vi "Arduino Analog Read Pin.vi"() -> ()   [LabVIEW 2011, in "LabVIEW Interface for Arduino.lvlib"]
doc: "An example that reads a user selectable analog input pin on the Arduino."
uses:
  <vilib>/LabVIEW Interface for Arduino/LabVIEW Interface for Arduino.lvlib
  <vilib>/LabVIEW Interface for Arduino/Type Defs/Analog Pin.ctl
panel:
  in  "Analog Pin":T1
  in  "Stop":bool
  out "Voltage":dbl(knob) scale=0.0..5.0
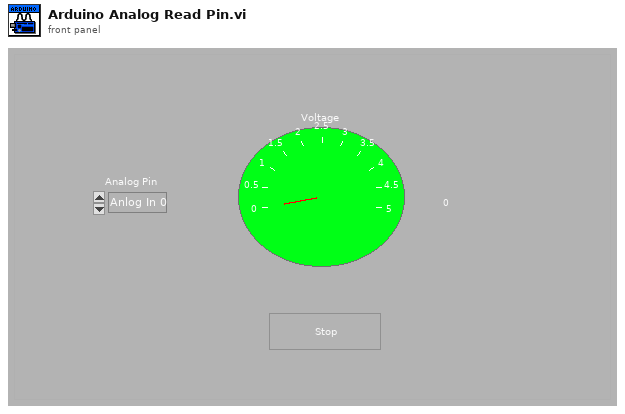
[diagram p1: front panel]
types:
  T1 = typedef "LabVIEW Interface for Arduino.lvlib/Analog Pin.ctl" = enum8{"Anlog In 0", "Anlog In 1", "Anlog In 2", "Anlog In 3", "Anlog In 4", "Anlog In 5"}
  T2 = typedef "LabVIEW Interface for Arduino.lvlib/Arduino Resource.ctl" = cluster{"VISA resource":refnum<visa-resource-name>, "Board Type":T3, "Connection Type":enum8{"USB / Serial"}, "Bytes Per Packet (15)":u8}
  T3 = typedef "LabVIEW Interface for Arduino.lvlib/Board Type.ctl" = enum16{"Uno", "Dimuelanove w/Atmega 328", "Mega 2560"}
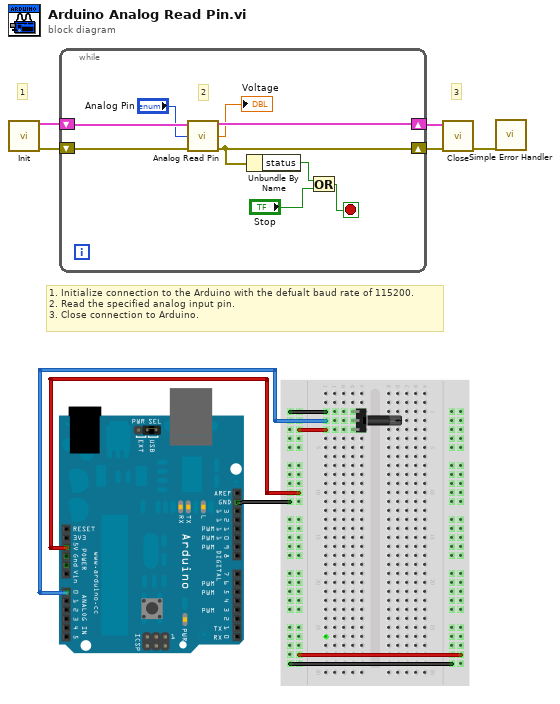
[diagram p0: block diagram]
diagram:
  # "1. Initialize connection to the Arduino with the defualt baud rate of 115200.\n2. Read the specified analog input pin.\n3. Close connection to Arduino."
  # "3"
  # "1"
  n1 = call <vilib>:"Init.vi"() -> ("Arduino Resource"=w5:T2, "error out"=w2:errorcluster)  [unwired: 18 in]
  n2 = while {
    shift-right: [w14] -> w4
    shift-left: w5 -> [w8]
    shift-right: [w12] -> w3
    shift-left: w2 -> [w7]
    stop <- w11 stop-if-true
    # "2"
    n3 = call <vilib>:"Analog Read Pin.vi"("Arduino Resource"=w8, "Analog Input Pin (0)"="Analog Pin", "error in"=w7) -> ("Arduino Resource"=w14:T2, "Voltage"=→"Voltage":dbl, "error out"=w12:errorcluster)  [unwired: 10 in]
    n4 = Unbundle By Name(w12) -> ("status"=w10:bool)
    n5 = Or(x=w10, y="Stop") -> (x .or. y?=w11:bool)
  }
  n6 = call <vilib>:"Close.vi"("Arduino Resource"=w4, "error in"=w3) -> ("error out"=w1:errorcluster)  [unwired: 13 in]
  n7 = call <vilib>:"Simple Error Handler.vi"("error in (no error)"=w1) -> ()  [unwired: 4 in, 5 out]
